vi "GEN40-38-LAN Identify.vi"(8 "error in (no error)":errorcluster, 10 "VISA resource name out":refnum<visa-resource-name>, 11 "GEN40-38-LAN in":refnum<class "GEN40-38-LAN.lvclass">) -> (0 "error out":errorcluster, 2 "Identification":T1, 3 "GEN40-38-LAN out":refnum<class "GEN40-38-LAN.lvclass">)   [LabVIEW 2018, in "GEN40-38-LAN.lvlib" / "GEN40-38-LAN.lvclass"]
doc: "This VI gets the Power Supply identification information and outputs the information in a cluster of 4 (four) components (Manufacturer, Model, Serial Number and Revisions)."
uses:
  GEN40-38-LAN.lvclass
  Custom Controls/Identification.ctl
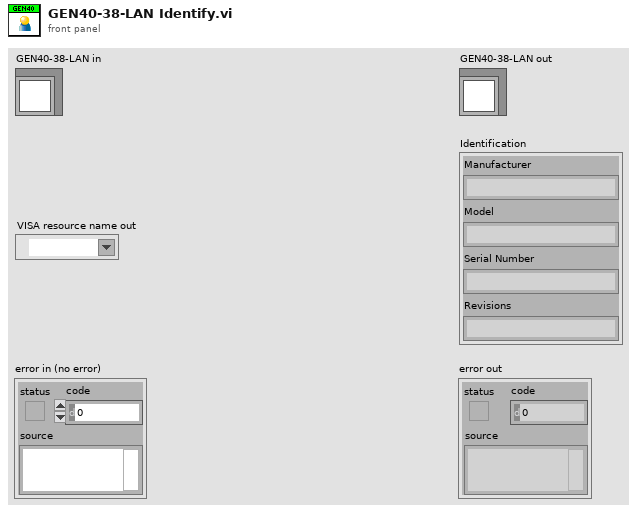
[diagram p1: front panel]
types:
  T1 = typedef "GEN40-38-LAN.lvlib/GEN40-38-LAN.lvclass/Identification.ctl" = cluster{"Manufacturer":string, "Model":string, "Serial Number":string, "Revisions":string}
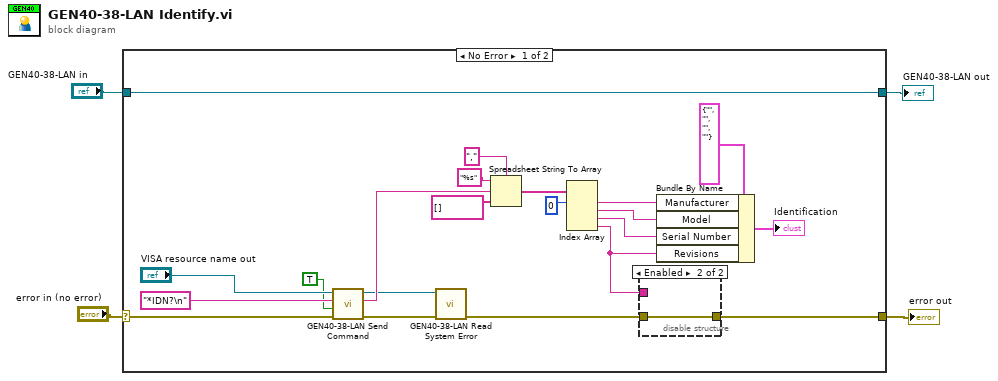
[diagram p0: block diagram]
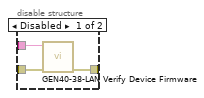
[diagram p2: hidden frame]
diagram:
  n1 = case shown="No Error" "error in (no error)" {
    selector: "error in (no error)" -> [w12 w31]
    tunnel: [w5 w31] -> w3
    tunnel: [w25 w30] -> w1
    tunnel: "GEN40-38-LAN in" -> [w25 w30]
    frame No Error {
      n2 = call "GEN40-38-LAN Send Command.vi"("error in (no error)"=w12, "Wait for Response?"=TRUE, "Command"="*IDN?\n" ("write buffer"), "VISA resource name"="VISA resource name out") -> ("error out"=w9:errorcluster, "Response"=w11:string, "VISA resource name out"=w8:refnum<visa-resource-name>)  [unwired: 5 in]
      n3 = call "GEN40-38-LAN Read System Error.vi"("error in (no error)"=w9, "Resource"=w8) -> ("error out"=w7:errorcluster)  [unwired: 9 in]
      n4 = Spreadsheet String To Array(delimiter (Tab)=",", format string="%s", spreadsheet string=w11, array type (2D Dbl)=string[] []) -> (array=w17:string[])
      n5 = Index Array(array=w17, index #1=0 ("index")) -> (element #1=w20:string, element #2=w21:string, element #3=w24:string, element #4=w6:string)  [unwired: 3 in]
      n6 = disable-structure shown="Enabled" {
        disable-tunnel: w7 -> [w28 w29]
        disable-tunnel: w6 -> [w27 _]
        disable-tunnel: [w26 w29] -> w5
        frame Disabled {
          n7 = call "GEN40-38-LAN Verify Device Firmware.vi"("error in"=w28, "Revisions"=w27) -> ("error out"=w26:errorcluster)  [unwired: 9 in]
        }
        frame Enabled {
        }
      }
      n8 = Bundle By Name(cluster=T1 {"Manufacturer"="", "Model"="", "Serial Number"="", "Revisions"=""} ("Identification"), "Manufacturer"=w20, "Model"=w21, "Serial Number"=w24, "Revisions"=w6) -> (→"Identification":T1)
    }
    frame Error {
    }
  }
  "error out" <- w3
  "GEN40-38-LAN out" <- w1
